vi "E517_Position.vi"() -> ()   [LabVIEW 2011]
panel:
  in  "POS X rad":dbl
  in  "POS Y rad":dbl
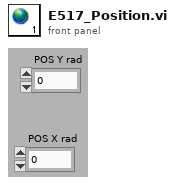
[diagram p1: front panel]
diagram:
